vi "LabVIEW Score Entry.vi"() -> (2 "Array":cluster{"Name":string, "Value":string}[](array[cluster]))   [LabVIEW 2013]
panel:
  in  "Penalties- Inside Light Blue":enum16{"[Null]", "0", "1", "2", "3", "4"}(ring)
  in  "Penalties- Outside Light Blue":enum16{"[Null]", "0", "1", "2", "3", "4"}(ring)
  in  "Safe Place":enum16{"[Null]", "Yes", "No"}(ring)
  in  "Supplies- In Yellow":T1(ring)
  in  "Supplies- In Red":T1(ring)
  in  "Pets":enum16{"[Null]", "0", "1", "2"}(ring)
  in  "Safety- People In Yellow":enum16{"[Null]", "0", "1", "2", "3"}(ring)
  in  "Safety- People In Red":enum16{"[Null]", "0", "1", "2", "3"}(ring)
  in  "Family":enum16{"[Null]", "None", "2", "3"}(ring)
  in  "Progress":enum16{"[Null]"}(ring)
  in  "Obstacles":T2(ring)
  in  "Code Construction":T3(ring)
  in  "Base Isolation":enum16{"[Null]", "Yes", "No"}(ring)
  in  "Construction Relocation":enum16{"[Null]", "Yes", "No"}(ring)
  in  "Runway Clear":enum16{"[Null]", "Yes", "No"}(ring)
  in  "Ambulance In Yellow":enum16{"[Null]", "Yes", "No"}(ring)
  in  "All Waves On Mat":enum16{"[Null]", "Yes", "No"}(ring)
  in  "Tree Branch Below Wires":enum16{"[Null]", "Yes", "No"}(ring)
  in  "Cargo Plane":enum16{"[Null]", "None", "Yellow", "Light Blue"}(ring)
  in  "Evac Sign Upright":enum16{"[Null]", "Yes", "No"}(ring)
  in  "Supply Truck On Yellow":enum16{"[Null]", "Yes", "No"}(ring)
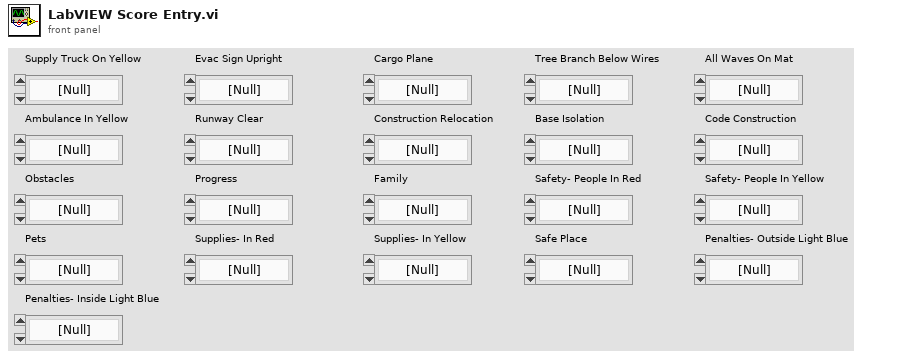
[diagram p1: front panel]
types:
  T1 = enum16{"[Null]", "0", "1", "2", "3", "4", "5", "6", "7", "8", "9", "10", "11", "12"}
  T2 = enum16{"[Null]", "None", "Dark Blue", "Dark Green", "Purple", "Red"}
  T3 = enum16{"[Null]", "0", "1", "2", "3", "4", "5", "6"}
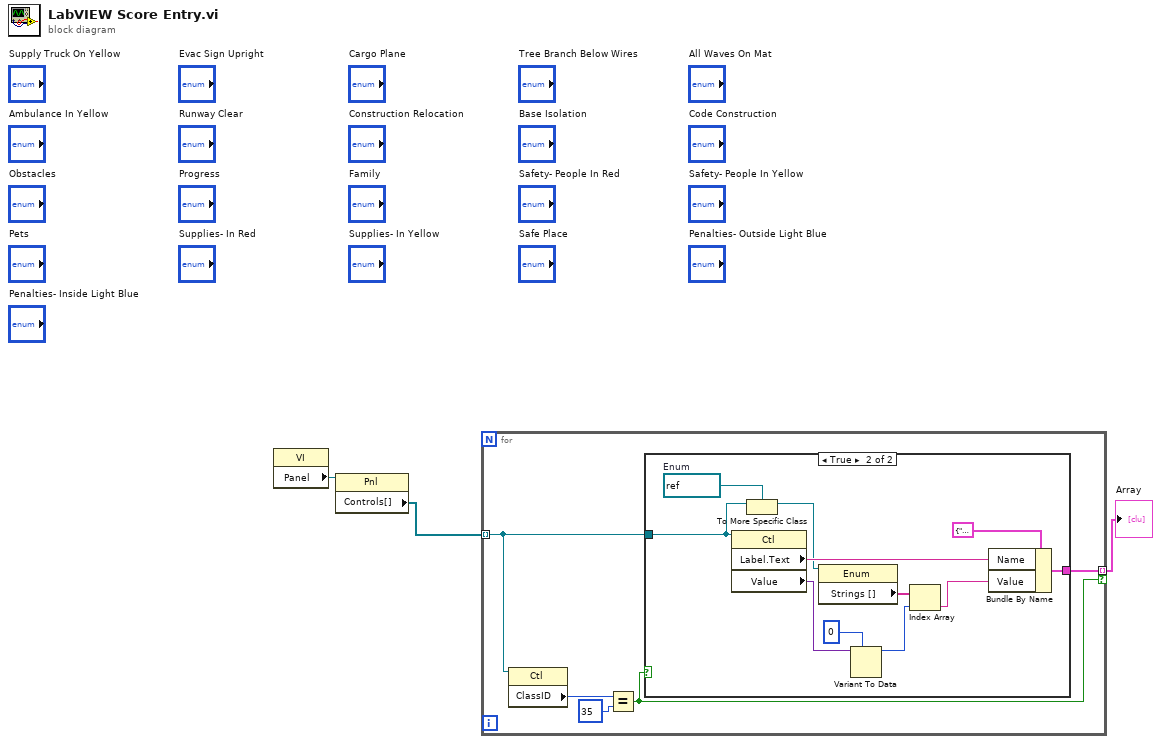
[diagram p0: block diagram]
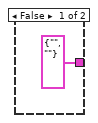
[diagram p2: hidden frame]
diagram:
  n1 = property class="VI"() -> ("Panel"=w3:refnum<vi>)  [unwired: 2 in, 2 out]
  n2 = property class="Pnl"(reference=w3) -> ("Controls[]"=w2:refnum<vi>[])  [unwired: 1 in, 2 out]
  n3 = for {
    tunnel: w2 -> [w7] mode=indexing
    tunnel: [w8] -> w1 mode=indexing if=w4
    n4 = property class="Ctl"(reference=w7) -> ("ClassID"=w6:u32)  [unwired: 1 in, 2 out]
    n5 = Equal?(x=w6, y=u32 35) -> (x = y?=w4:bool)
    n6 = case shown="True" w4 {
      tunnel: [cluster{"Name":string, "Value":string} {"Name"="", "Value"=""} w17] -> w8
      tunnel: w7 -> [_ w10]
      frame False {
      }
      frame True {
        w16 = refnum<vi> refnum  # Enum
        n7 = property class="Ctl"(reference=w10) -> ("Label.Text"=w18:string, "Value"=w20:variant)  [unwired: 1 in, 2 out]
        n8 = To More Specific Class(target class=w16, reference=w10) -> (specific class reference=w15:refnum<vi>)  [unwired: 1 in, 1 out]
        n9 = property class="Enum"(reference=w15) -> ("Strings []"=w13:string[])  [unwired: 1 in, 2 out]
        n10 = Variant To Data(type=u16 0, Variant=w20) -> (data=w12:u16)  [unwired: 1 in, 1 out]
        n11 = Index Array(array=w13, index=w12) -> (element=w11:string)
        n12 = Bundle By Name(cluster=cluster{"Name":string, "Value":string} {"Name"="", "Value"=""}, "Name"=w18, "Value"=w11) -> (w17:cluster{"Name":string, "Value":string})
      }
    }
  }
  "Array" <- w1
